vi "LibXML_ReplaceValue.vi"(6 "Node-Type":enum16{"Attribute", "Element"}(ring), 7 "Root-path (xpath)":string, 8 "error in":errorcluster, 9 "Name":string, 10 "New Value":string, 11 "doc":u32) -> (0 "error out":errorcluster, 3 "doc copy out":u32)   [LabVIEW 2019, in "Tools.lvlib" / "LibXML.lvlib"]
doc: "This vi searches values of attributes or elements in the given rootpath. If there ar more elements in the rootpath with the same name all values are found and put in the values-array. When only one value is expected (like in attributes) one can use the first value output.\nThe syntax for the rootpath is the XPath-syntax\nIf we want to find the values of the attribute\"axis\" of all ReadAxis elements under the ReadMethod element of the Datachannel with attribute name-id =\"Scan-data the root-path will be\n.//DataChannel[@name-id =\"Scan-data \"]/ReadMethod//ReadAxis\n while the name input should be axis, and the node type should be Attribute."
uses:
  LibXML.lvlib
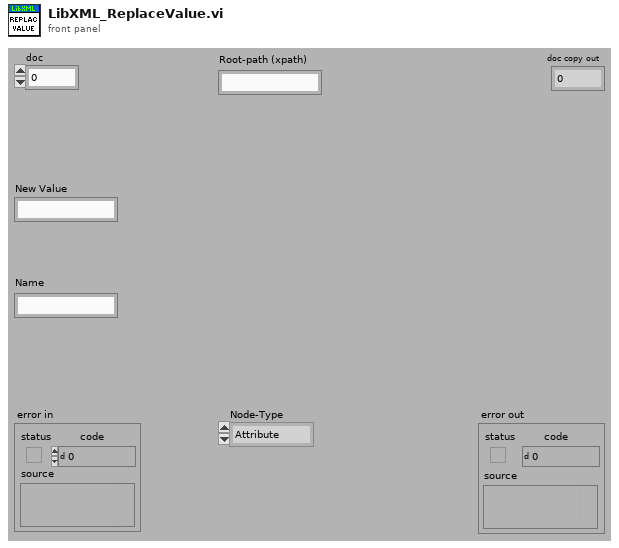
[diagram p1: front panel]
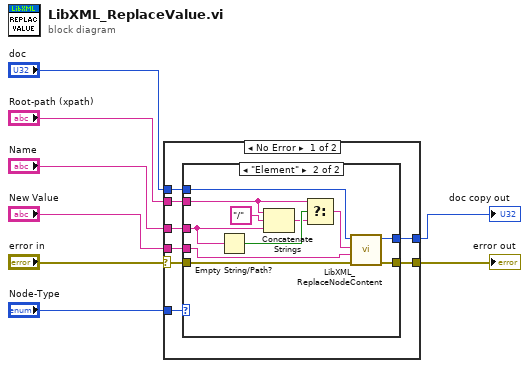
[diagram p0: block diagram]
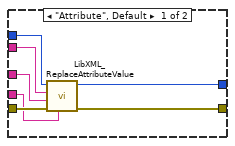
[diagram p2: hidden frame]
diagram:
  n1 = case shown="No Error" "error in" {
    selector: "error in" -> [w16 w36]
    tunnel: [w14 w36] -> w8
    tunnel: "doc" -> [w15 w35]
    tunnel: [w13 w35] -> w5
    tunnel: "Root-path (xpath)" -> [w12 _]
    tunnel: "Name" -> [w11 _]
    tunnel: "Node-Type" -> [w10 _]
    tunnel: "New Value" -> [w9 _]
    frame No Error {
      n2 = case shown="\"Element\"" w10 {
        tunnel: w12 -> [w20 w25]
        tunnel: w11 -> [w19 w24]
        tunnel: w16 -> [w23 w34]
        tunnel: w15 -> [w21 w32]
        tunnel: [w18 w31] -> w13
        tunnel: [w22 w30] -> w14
        tunnel: w9 -> [w17 w29]
        frame "Attribute", Default {
          n3 = call "LibXML_ReplaceAttributeValue.vi"("New Value"=w17, "error in"=w23, "attr. name"=w19, "xpathexpr (root)"=w20, "doc"=w21) -> ("error out"=w22:errorcluster, "doc copy out"=w18:u32)  [unwired: 5 in]
        }
        frame "Element" {
          n4 = Empty String/Path?(string/path=w24) -> (empty?=w27:bool)
          n5 = Concatenate Strings(w25, "/" ("string"), w24) -> (w26:string)
          n6 = Select(t=w25, s=w27, f=w26) -> (s? t:f=w33:string)
          n7 = call "LibXML_ReplaceNodeContent.vi"("error in"=w34, "New Value"=w29, "xpathexpr"=w33, "doc"=w32) -> ("error out"=w30:errorcluster, "doc copy out"=w31:u32)  [unwired: 6 in]
        }
      }
    }
    frame Error {
    }
  }
  "error out" <- w8
  "doc copy out" <- w5
